vi "set_update_owner_command.vi"(8 "error in (no error)":errorcluster, 10 "update-owner command":refnum<class "GenericImageProcessorChangedCommand.lvclass">, 11 "GenericImageProcessor.lvclass in":refnum<class "GenericImageProcessor.lvclass">) -> (0 "error out":errorcluster, 3 "GenericImageProcessor.lvclass out":refnum<class "GenericImageProcessor.lvclass">)   [LabVIEW 2010, in "GenericImageProcessor.lvclass"]
uses:
  GenericImageProcessor.lvclass
  Command/GenericImageProcessorChangedCommand/GenericImageProcessorChangedCommand/GenericImageProcessorChangedCommand.lvclass
  Command/GenericCommand/GenericCommand/GenericCommand.lvclass
  GenericImageProcessor.lvclass/GenericImageProcessor.ctl
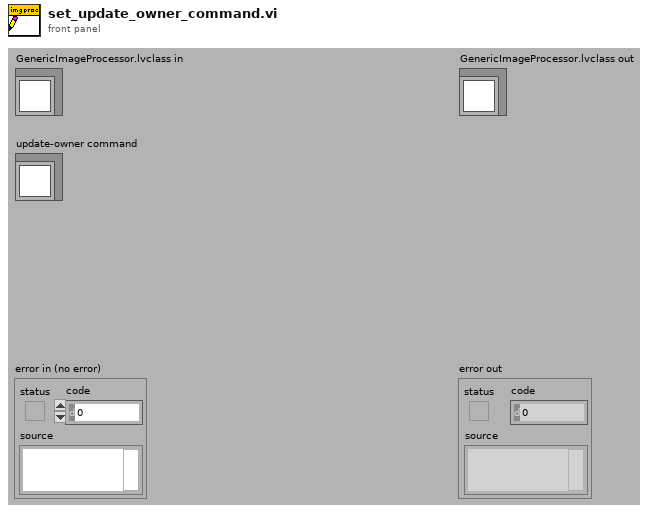
[diagram p1: front panel]
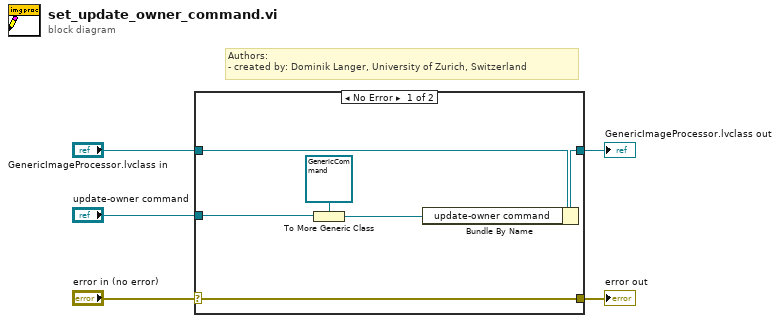
[diagram p0: block diagram]
diagram:
  # "Authors: \n- created by: Dominik Langer, University of Zurich, Switzerland"
  n1 = case shown="No Error" "error in (no error)" {
    selector: "error in (no error)" -> [w11 w12]
    tunnel: [w11 w12] -> w4
    tunnel: [w9 w13] -> w2
    tunnel: "GenericImageProcessor.lvclass in" -> [w10 w13]
    tunnel: "update-owner command" -> [w8 _]
    frame No Error {
      n2 = To More Generic Class(target class=refnum<class "GenericCommand.lvclass"> refnum ("GenericCommand.lvclass"), reference=w8) -> (generic class reference=w7:refnum<class "GenericCommand.lvclass">)
      n3 = Bundle By Name(cluster=w10, "update-owner command"=w7) -> (w9:refnum<class "GenericImageProcessor.lvclass">)
    }
    frame Error {
    }
  }
  "error out" <- w4
  "GenericImageProcessor.lvclass out" <- w2
